vi "Module API.vi"(8 "error in (no error)":errorcluster, 11 "DemoClass in":refnum<class "DemoClass.lvclass">) -> (0 "error out":errorcluster, 2 "API":refnum<class "API.lvclass">, 3 "DemoClass out":refnum<class "DemoClass.lvclass">)   [LabVIEW 2020]
uses:
  DemoClass.lvclass
  Volatus/API/API.lvclass
  DemoClass.lvclass/DemoClass.ctl
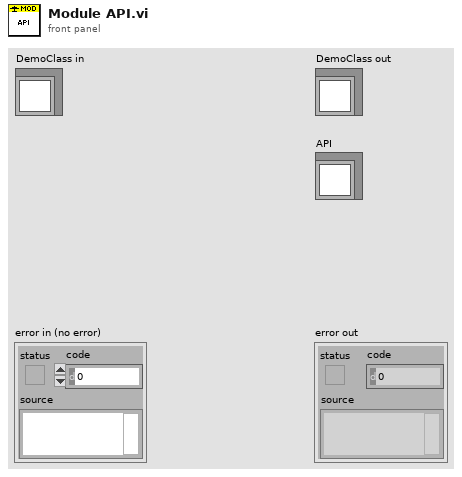
[diagram p1: front panel]
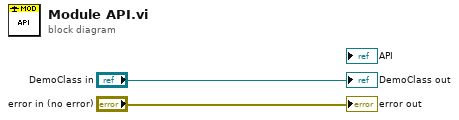
[diagram p0: block diagram]
diagram:
  "error out" <- "error in (no error)"
  "DemoClass out" <- "DemoClass in"
